vi "ReWrite Request.vi"(8 "error in":errorcluster, 11 "formdata":T1) -> (0 "error out":errorcluster)   [LabVIEW 2011]
uses:
  user project design.ctl
  Folders.ctl
  Design Server.lvlib
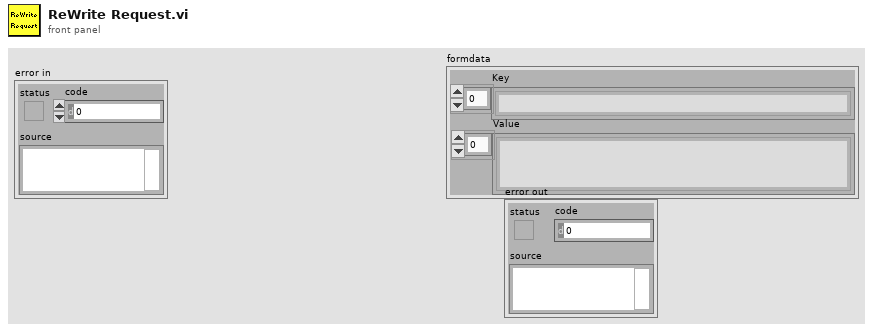
[diagram p1: front panel]
types:
  T1 = typedef "Design Server.lvlib/user project design.ctl" = cluster{"Key":string[], "Value":string[]}
  T2 = enum16{"open", "replace", "create", "open or create", "replace or create", "replace or create with confirmation"}
  T3 = typedef "Design Server.lvlib/Folders.ctl" = enum16{"MathcadMethods", "RequestedDesigns", "CompletedDesigns", "MathcadCode", "CollabnetSVN.exe"}
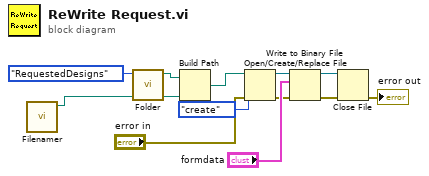
[diagram p0: block diagram]
diagram:
  n1 = call "Filenamer.vi"() -> ("Project Folder"=w1:path)  [unwired: 10 in, 1 out]
  n2 = call "Folder.vi"("Folders"=Folders."RequestedDesigns") -> ("FolderPath"=w11:path)  [unwired: 8 in, 2 out]
  n3 = Build Path(base path=w11, name or relative path=w1) -> (appended path=w9:path)
  n4 = Open/Create/Replace File(file path (use dialog)=w9, error in="error in", operation (0:open)=T2."create") -> (refnum out=w7:refnum<file>, error out=w6:errorcluster)  [unwired: 3 in, 1 out]
  n5 = Write to Binary File(file (use dialog)=w7, data="formdata", error in=w6) -> (refnum out=w4:refnum<file>, error out=w5:errorcluster)  [unwired: 3 in, 1 out]
  n6 = Close File(refnum=w4, error in=w5) -> (error out=→"error out":errorcluster)  [unwired: 1 out]
